vi "Letter to number.vi"(11 "String":string) -> (3 "Number":i32)   [LabVIEW 2015]
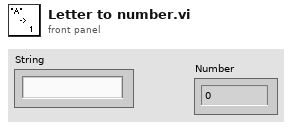
[diagram p1: front panel]
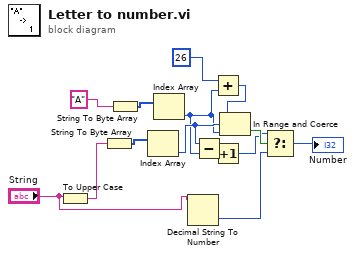
[diagram p0: block diagram]
diagram:
  n1 = To Upper Case(1:"String") -> (0:w14:string)
  n2 = String To Byte Array(string=w14) -> (unsigned byte array=w13:u8[])
  n3 = String To Byte Array(string="A") -> (unsigned byte array=w12:u8[])
  n4 = Index Array(array=w13) -> (element=w3:u8)  [unwired: 1 in]
  n5 = Index Array(array=w12) -> (element=w2:u8)  [unwired: 1 in]
  n6 = Decimal String To Number(string="String") -> (number=w6:i32)  [unwired: 2 in, 1 out]
  n7 = Subtract(x=w3, y=w2) -> (x-y=w4:u8)
  n8 = Add(x=u8 26, y=w2) -> (x+y=w9:u8)
  n9 = Increment(x=w4) -> (x+1=w1:u8)
  n10 = In Range and Coerce(upper limit=w9, x=w3, lower limit=w2) -> (In Range?=w8:bool)  [unwired: 1 out]
  n11 = Select(t=w1, s=w8, f=w6) -> (s? t:f=→"Number":i32)
